vi "FdxSubIrigStructIrigCvi.vi"(8 "error in":errorcluster, 11 "IRIG IN A/B":T2) -> (0 "error out":errorcluster, 3 "IRIG OUT":T1)   [LabVIEW 2020, in "AIM664LV.lvlib"]
doc: "This function is used to calculate time tag diffrences. \nResult = IRIG Time A - IRIG Time B (sub)\n(Calculates with 366 Days / Year)"
uses:
  AIM664LV.lvlib
  AFDX_LibraryAdmin/FdxGlobalDllPath.vi
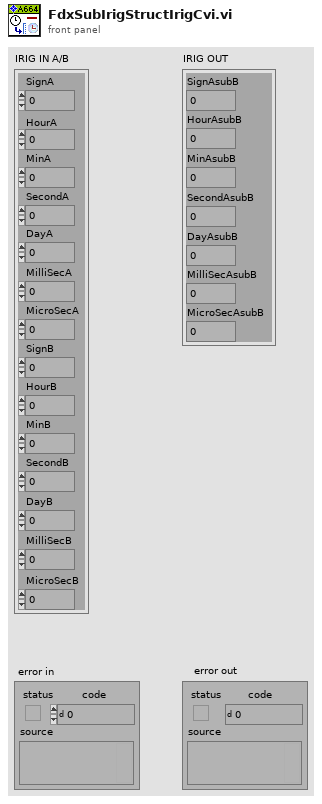
[diagram p1: front panel]
types:
  T1 = cluster{"SignAsubB":i32, "HourAsubB":u32, "MinAsubB":u32, "SecondAsubB":u32, "DayAsubB":u32, "MilliSecAsubB":u32, "MicroSecAsubB":u32}
  T2 = cluster{"SignA":i32, "HourA":u32, "MinA":u32, "SecondA":u32, "DayA":u32, "MilliSecA":u32, "MicroSecA":u32, "SignB":i32, "HourB":u32, "MinB":u32, "SecondB":u32, "DayB":u32, "MilliSecB":u32, "MicroSecB":u32}
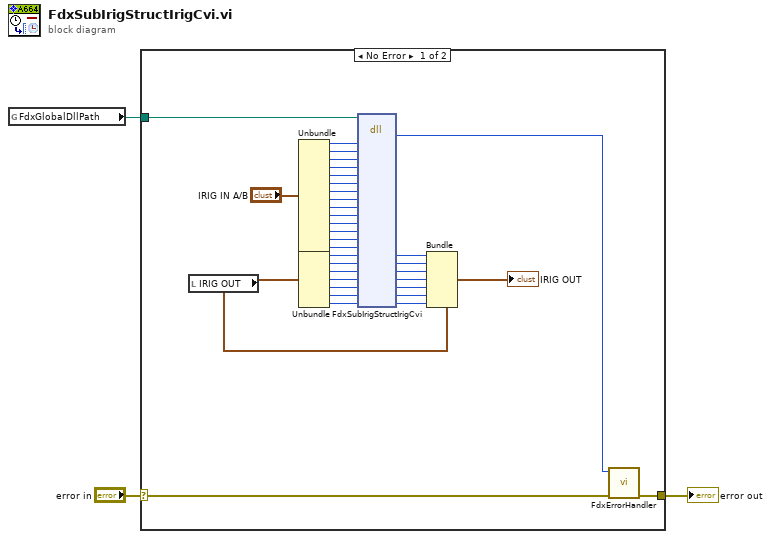
[diagram p0: block diagram]
diagram:
  n1 = global read "FdxGlobalDllPath.vi" "FdxGlobalDllPath"() -> (w1:path)
  n2 = case shown="No Error" "error in" {
    selector: "error in" -> [w37 w39]
    tunnel: [w38 w39] -> w3
    tunnel: w1 -> [w4 _]
    frame No Error {
      n3 = local read "IRIG OUT"() -> (w12:T1)
      n4 = Unbundle("IRIG IN A/B") -> ("SignA"=w29:i32, "HourA"=w28:u32, "MinA"=w27:u32, "SecondA"=w26:u32, "DayA"=w25:u32, "MilliSecA"=w24:u32, "MicroSecA"=w23:u32, "SignB"=w22:i32, "HourB"=w21:u32, "MinB"=w20:u32, "SecondB"=w19:u32, "DayB"=w18:u32, "MilliSecB"=w17:u32, "MicroSecB"=w16:u32)
      n5 = Unbundle(w12) -> ("SignAsubB"=w11:i32, "HourAsubB"=w10:u32, "MinAsubB"=w9:u32, "SecondAsubB"=w8:u32, "DayAsubB"=w7:u32, "MilliSecAsubB"=w6:u32, "MicroSecAsubB"=w5:u32)
      n6 = dll-call lib="aim_fdx.19.dll" fn="FdxSubIrigStructIrigCvi"(path in=w4, "SignA"=w29, "HourA"=w28, "MinA"=w27, "SecondA"=w26, "DayA"=w25, "MilliSecA"=w24, "MicroSecA"=w23, "SignB"=w22, "HourB"=w21, "MinB"=w20, "SecondB"=w19, "DayB"=w18, "MilliSecB"=w17, "MicroSecB"=w16, "SignAsubB"=w11, "HourAsubB"=w10, "MinAsubB"=w9, "SecondAsubB"=w8, "DayAsubB"=w7, "MilliSecAsubB"=w6, "MicroSecAsubB"=w5) -> ("status"=w36:i32, "SignAsubB"=w30:i32, "HourAsubB"=w31:u32, "MinAsubB"=w32:u32, "SecondAsubB"=w33:u32, "DayAsubB"=w15:u32, "MilliSecAsubB"=w14:u32, "MicroSecAsubB"=w13:u32)  [unwired: 16 in, 2 out]
      n7 = Bundle(cluster=w12, "SignAsubB"=w30, "HourAsubB"=w31, "MinAsubB"=w32, "SecondAsubB"=w33, "DayAsubB"=w15, "MilliSecAsubB"=w14, "MicroSecAsubB"=w13) -> (→"IRIG OUT":T1)
      n8 = call "FdxErrorHandler.vi"("error in"=w37, "AIM Error"=w36) -> ("error out"=w38:errorcluster)  [unwired: 9 in]
    }
    frame Error {
    }
  }
  "error out" <- w3
